vi "CrossCorrelationFFT.vi"(2 "Input 2":fxp<+/-,24,8>, 3 "Input 1":fxp<+/-,24,8>) -> (0 "Index":u16, 1 "Cross Correlation":fxp<+/-,32,16>)   [LabVIEW 2015]
uses:
  <vilib>/rvi/Analysis/measure/FFT/simModelSupport/niFPGA FFT Outside SCTL Sim Properties.ctl
  <vilib>/rvi/Analysis/measure/FFT/simModelSupport/niFPGA FFT Sim Types.ctl
  <vilib>/rvi/Analysis/measure/FFT/simModelSupport/niFpgaFFTSimArithmeticProperties.ctl
  <vilib>/rvi/Analysis/measure/FFT/simModelSupport/niFpgaFFTSimDfxp.ctl
  <vilib>/fxp/LVFixedPointQuantizationPolicyTypeDef.ctl
  <vilib>/rvi/FXPMathLib/SharedSubVIs/typedef/nifxpmath_BASIC_ImplementationSettings.ctl
  <vilib>/fxp/LVFixedPointOverflowPolicyTypeDef.ctl
  <vilib>/rvi/ClientSDK/Core/DevComputerLib/Private/Dfxp64.ctl
  <vilib>/fxp/LVFixedPointRepBitsTypeDef.ctl
  <vilib>/rvi/ClientSDK/Core/DevComputerLib/Private/Dfxp64OutputConfig.ctl
  <vilib>/rvi/Analysis/measure/FFT/simModelSupport/niFpgaFFTSimModelOutsideSCTLCore.vi
  <vilib>/rvi/ClientSDK/Core/DevComputerLib/Private/ComplexMultiply(dfxp64).vi
  <vilib>/rvi/ClientSDK/Core/DevComputerLib/Private/FourWireProtocol(cint64).vi
  <vilib>/rvi/Analysis/measure/FFT/XNode/niFpgaFFT.xnode
  <vilib>/rvi/FXPMathLib/FxpMultComplex/XNode/niFpgaMultComplex.xnode
  <vilib>/rvi/ClientSDK/Core/DevComputerLib/niFpgaDevCompUtilities.lvlib
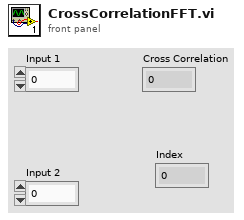
[diagram p1: front panel]
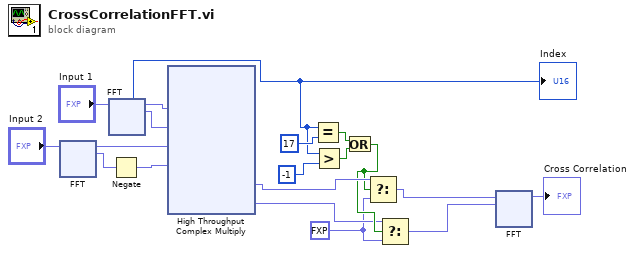
[diagram p0: block diagram]
diagram:
  w2 = fxp<+/-,32,16> 0.0
  n1 = xnode "FFT"("real data in"="Input 2") -> ("real data out"=w16:fxp<+/-,32,19>, "imaginary data out"=w17:fxp<+/-,32,19>)  [unwired: 2 in, 1 out]
  n2 = xnode "FFT"("real data in"="Input 1") -> ("data index"=w8:u16, "real data out"=w14:fxp<+/-,32,19>, "imaginary data out"=w15:fxp<+/-,32,19>)  [unwired: 2 in]
  "Index" <- w8
  n3 = Negate(x=w17) -> (-x=w18:fxp<+/-,33,20>)
  n4 = xnode ("High Throughput Complex Multiply")("xr"=w14, "xi"=w15, "yr"=w16, "yi"=w18) -> ("pr"=w6:fxp<+/-,32,15>, "pi"=w3:fxp<+/-,32,15>)
  n5 = Equal?(x=w8, y=u32 17) -> (x = y?=w10:bool)
  n6 = Greater?(x=w8, y=-1) -> (0:w9:bool)
  n7 = Or(x=w10, y=w9) -> (x .or. y?=w4:bool)
  n8 = Select(t=w6, s=w4, f=w2) -> (s? t:f=w5:fxp<+/-,33,16>)
  n9 = Select(t=w3, s=w4, f=w2) -> (s? t:f=w1:fxp<+/-,33,16>)
  n10 = xnode "FFT"("real data in"=w5, "imaginary data in"=w1) -> ("real data out"=→"Cross Correlation":fxp<+/-,32,17>)  [unwired: 1 in, 2 out]
